vi "GetAppOutput.vi"(8 "error in (no error)":errorcluster, 11 "LSEPlugin in":refnum<class "LSEPlugin.lvclass">) -> (0 "error out":errorcluster, 3 "LSEPlugin out":refnum<class "LSEPlugin.lvclass">)   [LabVIEW 2014, in "AppPlugins.lvlib" / "LSEPlugin.lvclass"]
uses:
  LSEPlugin.lvclass
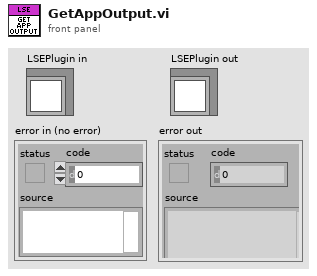
[diagram p1: front panel]
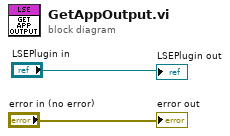
[diagram p0: block diagram]
diagram:
  "error out" <- "error in (no error)"
  "LSEPlugin out" <- "LSEPlugin in"
